vi "Enable_Disable.vi"(0 "Set Pin Status":refnum<vi>, 1 "Get Pin Status":refnum<vi>, 2 "Set Port Status":refnum<vi>, 3 "Get Port Status":refnum<vi>, 4 "Read ADC":refnum<vi>, 5 "Byte 0":refnum<vi>, 6 "Byte 1":refnum<vi>, 9 "Valor pin":refnum<vi>, 11 "PIN":refnum<vi>, 12 "Fallo en conexion":bool, 13 "CH":refnum<vi>, 15 "Display":refnum<vi>) -> ()   [LabVIEW 2020, in "UI Actor.lvlib" / "UI Actor.lvclass"]
doc: "Habilita o desabilta dependiendo la conexión"
uses:
  UI Actor.lvclass
panel:
  in  "ComboBox in":refnum<vi>
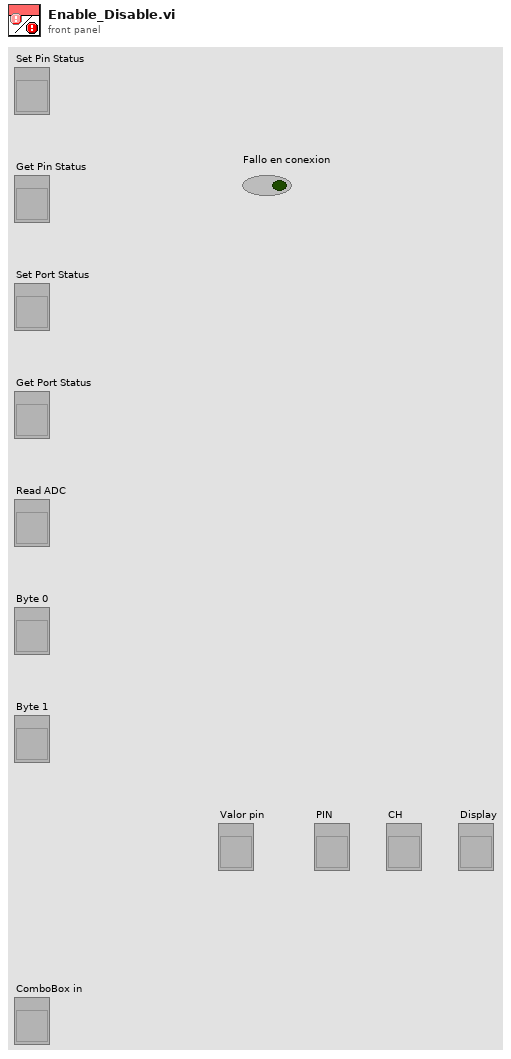
[diagram p1: front panel]
types:
  T1 = enum8{"Enabled", "Disabled", "Disabled and Grayed Out"}
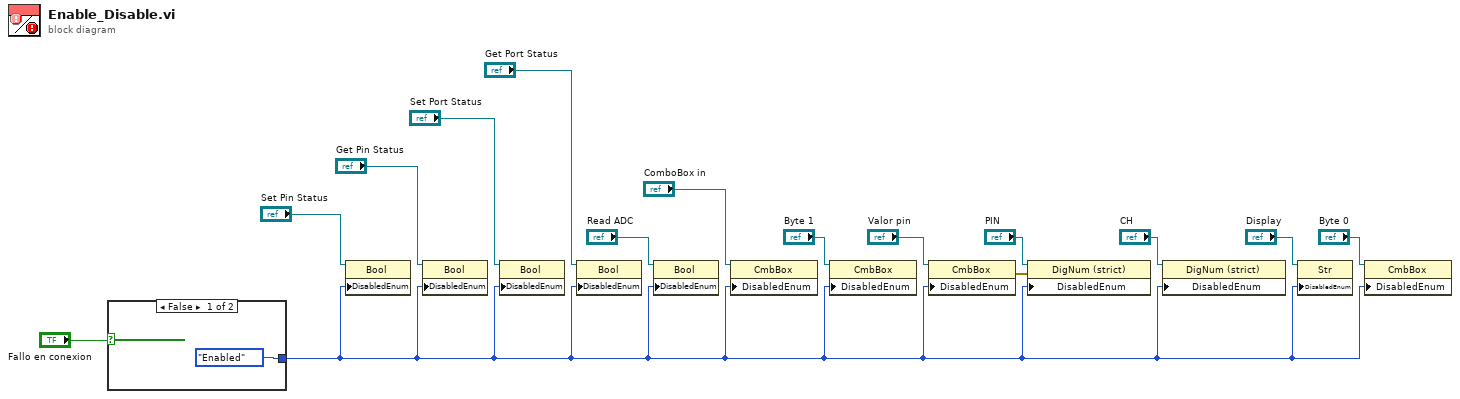
[diagram p0: block diagram]
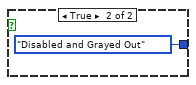
[diagram p2: hidden frame]
diagram:
  n1 = case shown="False" "Fallo en conexion" {
    tunnel: [T1."Enabled" ("Disabled") T1."Disabled and Grayed Out" ("Disabled")] -> w3
    frame False {
    }
    frame True {
    }
  }
  n2 = property class="Bool"(reference="Set Pin Status", "DisabledEnum"=w3) -> ()  [unwired: 1 in, 2 out]
  n3 = property class="Bool"(reference="Get Pin Status", "DisabledEnum"=w3) -> ()  [unwired: 1 in, 2 out]
  n4 = property class="Bool"(reference="Set Port Status", "DisabledEnum"=w3) -> ()  [unwired: 1 in, 2 out]
  n5 = property class="Bool"(reference="Get Port Status", "DisabledEnum"=w3) -> ()  [unwired: 1 in, 2 out]
  n6 = property class="Bool"(reference="Read ADC", "DisabledEnum"=w3) -> ()  [unwired: 1 in, 2 out]
  n7 = property class="CmbBox"(reference="ComboBox in", "DisabledEnum"=w3) -> ()  [unwired: 1 in, 2 out]
  n8 = property class="CmbBox"(reference="Byte 1", "DisabledEnum"=w3) -> ()  [unwired: 1 in, 2 out]
  n9 = property class="CmbBox"(reference="Valor pin", "DisabledEnum"=w3) -> (error out=w4:errorcluster)  [unwired: 1 in, 1 out]
  n10 = property class="DigNum (strict)"(reference="PIN", error in=w4, "DisabledEnum"=w3) -> ()  [unwired: 2 out]
  n11 = property class="DigNum (strict)"(reference="CH", "DisabledEnum"=w3) -> ()  [unwired: 1 in, 2 out]
  n12 = property class="Str"(reference="Display", "DisabledEnum"=w3) -> ()  [unwired: 1 in, 2 out]
  n13 = property class="CmbBox"(reference="Byte 0", "DisabledEnum"=w3) -> ()  [unwired: 1 in, 2 out]
